vi "SPD.AP Meas Const T.vi"(5 "Continue":refnum<vi>, 6 "Temperature index":i32, 7 "Progress":refnum<vi>, 8 "Error In":errorcluster, 10 "APParams":T1, 11 "SPD.Stand Ctrl in":T2 {"spdDeviceSession"."hidSPD.Sturtup Values"."HV_bias" format="%#_6p, V"; "spdDeviceSession"."hidSPD.Sturtup Values"."TSet" format="%#_6p, DegC"; "spdDeviceSession"."hidSPD.Controller"."HV_bias" format="%#_6p, V"; "spdDeviceSession"."hidSPD.Controller"."TSet" format="%#_6p, DegC"}) -> (0 "Error Out":errorcluster, 1 "pass":bool, 2 "Report":string, 3 "SPD.Stand Ctrl out":T2 {"spdDeviceSession"."hidSPD.Sturtup Values"."HV_bias" format="%#_6p, V"; "spdDeviceSession"."hidSPD.Sturtup Values"."TSet" format="%#_6p, DegC"; "spdDeviceSession"."hidSPD.Controller"."HV_bias" format="%#_6p, V"; "spdDeviceSession"."hidSPD.Controller"."TSet" format="%#_6p, DegC"})   [LabVIEW 2018]
uses:
  typedefs/SPD.Stand Ctrl.ctl
  Instruments/SPD HID Interface/hidSPDLibForLabView/LibVIs/hidSPD Controls/hidSPD Device Session.ctl
  Instruments/SPD HID Interface/hidSPDLibForLabView/LibVIs/hidSPD Controls/hidSPD Controller.ctl
  Instruments/SPD HID Interface/hidSPDLibForLabView/LibVIs/hidSPD Controls/hidSPD SPD Type.ctl
  Instruments/KC705 DevBoard/typedefs/DevB.Session.ctl
  Instruments/KeySight 53230A/typedefs/FreqC.Session.ctl
  Instruments/KeySight 8164B/KeySight 8164B LAN InstrLib/typedefs/KeySight 8164B control.ctl
  Instruments/LeCroy SDA830/typedefs/LeCroy.Session.ctl
  typedefs/SPD.Events.ctl
  ConfigFile/SPD.Config File ctrl.ctl
  <vilib>/Utility/config.llb/Config Data RefNum.ctl
  typedefs/SPD.Meas Result.ctl
  typedefs/SPD.Queues.ctl
  typedefs/SPD.Stand state.ctl
  typedefs/SPD.AP Test Params.ctl
  typedefs/SPD.QE Strobe_Phase Tune Limits.ctl
  Instruments/KeySight 8164B/KeySight 8164B LAN InstrLib.lvlib
  <vilib>/Utility/config.llb/NI_LVConfig.lvlib
  Instruments/SPD HID Interface/hidSPDLibForLabView/hidSPDLibForLabView.lvlib
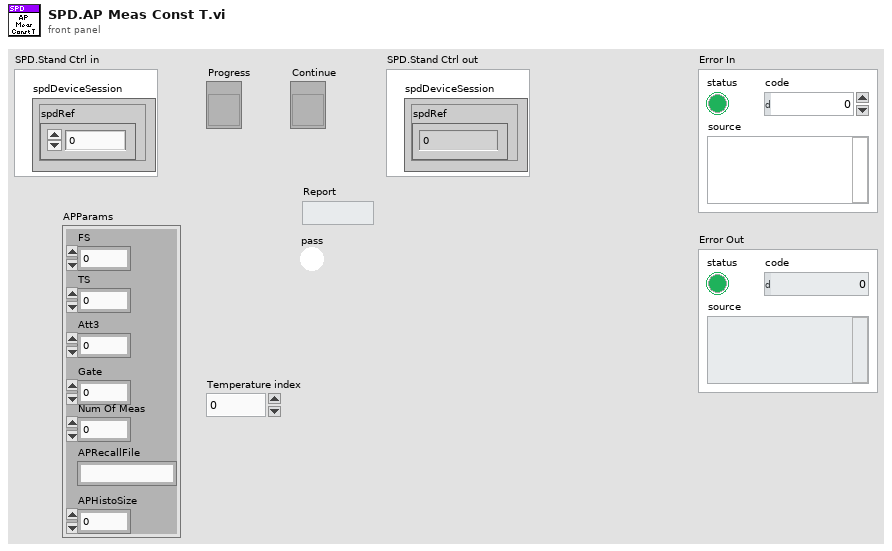
[diagram p1: front panel]
types:
  T1 = typedef "SPD.AP Test Params.ctl" = cluster{"FS":i32, "TS":i32, "Att3":dbl, "Gate":dbl, "Num Of Meas":i32, "APRecallFile":string, "APHistoSize":i32}
  T2 = typedef "SPD.Stand Ctrl.ctl" = cluster{"spdDeviceSession":T3, "DevBSession":T6, "FreqCSession":T7, "8164BSession":T8, "LeCroySession":T9, "Events":T10, "configFile":T11, "SPD.Result":T13, "SPD.Queues":T14, "Console":refnum<vi>}
  T3 = typedef "hidSPDLibForLabView.lvlib/hidSPD Device Session.ctl" = cluster{"spdRef":u64, "connected":bool, "spdName":string, "hidSPD.Controller":T4, "hidSPD.Sturtup Values":T4, "SPD Type":T5}
  T4 = typedef "hidSPDLibForLabView.lvlib/hidSPD Controller.ctl" = cluster{"TSet":sgl, "HV_bias":sgl, "DDS_stb_code":u16}
  T5 = typedef "hidSPDLibForLabView.lvlib/hidSPD SPD Type.ctl" = enum16{"Free Run", "Gate"}
  T6 = typedef "DevB.Session.ctl" = cluster{"DevBRef":refnum<visa-resource-name>, "connected":bool}
  T7 = typedef "FreqC.Session.ctl" = cluster{"FreqCRef":refnum<visa-resource-name>, "timeout":dbl, "Gate":dbl, "connected":bool}
  T8 = typedef "KeySight 8164B LAN InstrLib.lvlib/KeySight 8164B control.ctl" = cluster{"Connection ID":refnum<k5>, "Connected":bool, "Info":string, "Slots Info":string[]}
  T9 = typedef "LeCroy.Session.ctl" = cluster{"LeCroySession":refnum<visa-resource-name>, "connected":bool}
  T10 = typedef "SPD.Events.ctl" = cluster{"DCRTest":refnum<user-event>, "Stop":refnum<user-event>}
  T11 = typedef "SPD.Config File ctrl.ctl" = cluster{"configFile ref":T12, "configFile path":path, "equipmentFile ref":T12}
  T12 = typedef "NI_LVConfig.lvlib/Config Data RefNum.ctl" = refnum<k1>
  T13 = typedef "SPD.Meas Result.ctl" = cluster{"HV_Bias":dbl[][][], "Stb_code":dbl[], "Temprature":dbl[], "Data":dbl[][][][], "DateTime":string}
  T14 = typedef "SPD.Queues.ctl" = cluster{"state queue":refnum<queue>}
  T15 = typedef "SPD.QE Strobe_Phase Tune Limits.ctl" = cluster{"ph_start":i32, "ph_stop":i32, "ph_step":i32}
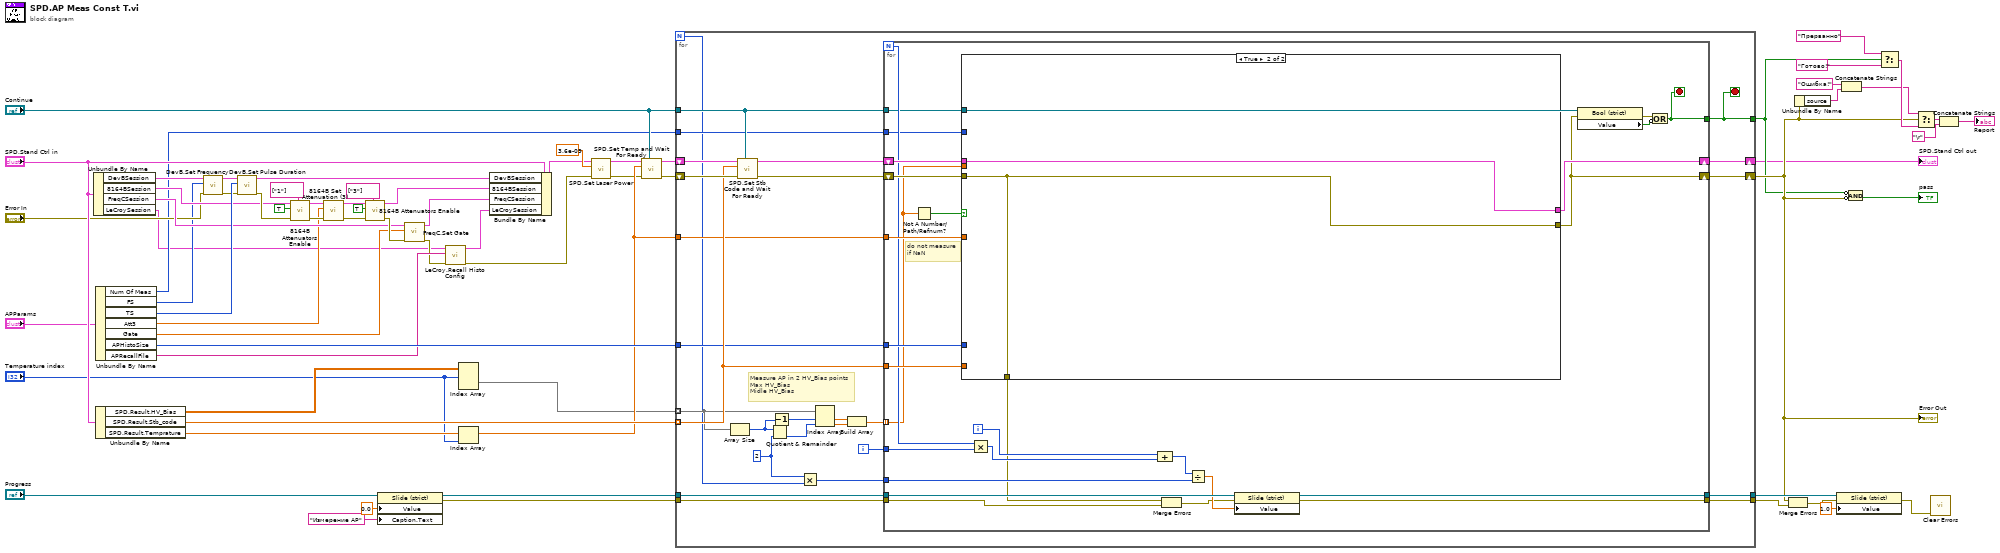
[diagram p0: block diagram]
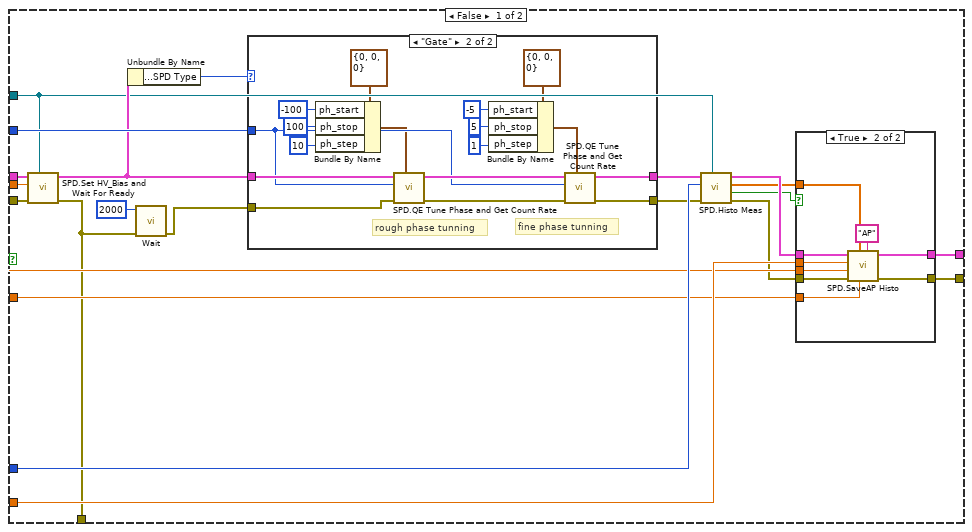
[diagram p2: hidden frame]
diagram:
  n1 = Unbundle By Name("SPD.Stand Ctrl in") -> ("DevBSession"=w61:T6, "8164BSession"=w51:T8, "FreqCSession"=w50:T7, "LeCroySession"=w7:T9)
  n2 = Unbundle By Name("APParams") -> ("Num Of Meas"=w38:i32, "FS"=w36:i32, "TS"=w59:i32, "Att3"=w37:dbl, "Gate"=w39:dbl, "APHistoSize"=w23:i32, "APRecallFile"=w9:string)
  n3 = Unbundle By Name("SPD.Stand Ctrl in") -> ("SPD.Result.HV_Bias"=w62:dbl[][][], "SPD.Result.Stb_code"=w63:dbl[], "SPD.Result.Temprature"=w64:dbl[])
  n4 = call "DevB.Set Frequency.vi"("error in (no error)"="Error In", "Frequency"=w36, "DevB Session in"=w61) -> ("error out"=w58:errorcluster, "DevB Session out"=w60:T6)  [unwired: 7 in]
  n5 = call "DevB.Set Pulse Duration.vi"("error in (no error)"=w58, "Pulse Duration"=w59, "DevB Session in"=w60) -> ("error out"=w53:errorcluster, "DevB Session out"=w49:T6)  [unwired: 7 in]
  n6 = call "8164B Attenuators Enable.vi"("Slots"=string[] ["1"], "error in"=w53, "Enable"=TRUE, "KeySight 8164B control in"=w51) -> ("error out"=w41:errorcluster, "KeySight 8164B control out"=w43:T8)  [unwired: 6 in]
  n7 = call "8164B Set Attenuation (3).vi"("error in"=w41, "Att 3, dB"=w37, "KeySight 8164B control in"=w43) -> ("error out"=w40:errorcluster, "KeySight 8164B control out"=w42:T8)  [unwired: 7 in]
  n8 = call "8164B Attenuators Enable.vi"("Slots"=string[] ["3"], "error in"=w40, "Enable"=TRUE, "KeySight 8164B control in"=w42) -> ("error out"=w52:errorcluster, "KeySight 8164B control out"=w48:T8)  [unwired: 6 in]
  n9 = property class="Slide (strict)"(reference="Progress", "Value"=0.0, "Caption.Text"="Измерение AP") -> (reference out=w15:refnum<vi>, error out=w13:errorcluster)  [unwired: 1 in]
  n10 = call "FreqC.Set Gate.vi"("error In"=w52, "Gate, sec"=w39, "FreqC Session in"=w50) -> ("error out"=w8:errorcluster, "FreqC Session out"=w47:T7)  [unwired: 7 in]
  n11 = call "LeCroy.Recall Histo Config.vi"("Error In"=w8, "Filename (panel.lss)"=w9, "LeCroy.Session in"=w7) -> ("Error Out"=w2:errorcluster, "LeCroy.Session out"=w6:T9)  [unwired: 7 in]
  n12 = Index Array(array=w62, index (dim 0)="Temperature index") -> (element=w18:dbl[][])  [unwired: 2 in]
  n13 = Index Array(array=w64, index="Temperature index") -> (element=w19:dbl)
  n14 = Bundle By Name(cluster="SPD.Stand Ctrl in", "DevBSession"=w49, "8164BSession"=w48, "FreqCSession"=w47, "LeCroySession"=w6) -> (w4:T2)
  n15 = call "SPD.Set Laser Power.vi"("Error In"=w2, "Pset"=3.6e-09, "SPD.Stand Ctrl in"=w4) -> ("Error Out"=w1:errorcluster, "SPD.Stand Ctrl out"=w3:T2)  [unwired: 7 in]
  n16 = call "SPD.Set Temp and Wait For Ready.vi"("Continue"="Continue", "Error In"=w1, "Tset"=w19, "SPD.Stand Ctrl in"=w3) -> ("Error Out"=w21:errorcluster, "SPD.Stand Ctrl out"=w20:T2)  [unwired: 6 in]
  n17 = for {
    N -> [w71]
    tunnel: w18 -> [w84] mode=indexing
    tunnel: w63 -> [w87] mode=indexing
    shift-right: [w95] -> w22
    shift-left: w20 -> [w93]
    shift-right: [w94] -> w26
    shift-left: w21 -> [w92]
    tunnel: "Continue" -> [w77]
    tunnel: [w90] -> w25
    tunnel: w15 -> [w89]
    tunnel: [w88] -> w67
    tunnel: w38 -> [w76]
    tunnel: w23 -> [w86]
    tunnel: w19 -> [w85]
    tunnel: w13 -> [w70]
    tunnel: [w69] -> w11
    i -> [w91]
    stop <- w90 stop-if-true
    w72 = 2 ("y")
    # "Measure AP in 2 HV_Bias points\nMax HV_Bias \nMidle HV_Bias"
    n18 = Array Size(array=w84) -> (size(s)=w82:i32)
    n19 = call "SPD.Set Stb Code and Wait For Ready.vi"("Continue"=w77, "Error In"=w92, "Strobe code"=w87, "SPD.Stand Ctrl in"=w93) -> ("Error Out"=w74:errorcluster, "SPD.Stand Ctrl out"=w75:T2)  [unwired: 6 in]
    n20 = Quotient & Remainder(x=w82, y=w72) -> (floor(x/y)=w83:i32)  [unwired: 1 out]
    n21 = Decrement(x=w82) -> (x-1=w81:i32)
    n22 = Multiply(x=w72, y=w71) -> (x*y=w73:i32)
    n23 = Index Array(array=w84, index #1=w81, index #2=w83) -> (element #1=w80:dbl, element #2=w79:dbl)
    n24 = Build Array(w80, w79) -> (w78:dbl[])
    n25 = for {
      N -> [w105]
      tunnel: w78 -> [w96] mode=indexing
      shift-right: [w108] -> w95
      shift-left: w75 -> [w122]
      shift-right: [w107] -> w94
      shift-left: w74 -> [w121]
      tunnel: w77 -> [w99]
      tunnel: w91 -> [w111]
      tunnel: [w118] -> w90
      tunnel: w89 -> [w117]
      tunnel: w73 -> [w115]
      tunnel: [w113] -> w88
      tunnel: w76 -> [w103]
      tunnel: w87 -> [w109]
      tunnel: w86 -> [w110]
      tunnel: w85 -> [w106]
      tunnel: w70 -> [w101]
      tunnel: [w100] -> w69
      i -> [w104]
      stop <- w118 stop-if-true
      # "do not measure\nif NaN"
      n26 = Not A Number/Path/Refnum?(number/path/refnum=w96) -> (NaN/Path/Refnum?=w97:bool)
      n27 = case shown="True" w97 {
        tunnel: w122 -> [w143 w175]
        tunnel: w121 -> [w142 w174]
        tunnel: w110 -> [w141 _]
        tunnel: w109 -> [w140 _]
        tunnel: w96 -> [w139 _]
        tunnel: [w138 w175] -> w108
        tunnel: [w137 w174] -> w107
        tunnel: w106 -> [w136 _]
        tunnel: w103 -> [w130 _]
        tunnel: w99 -> [w127 _]
        tunnel: [w125 w174] -> w98
        frame False {
          n28 = call "SPD.Set HV_Bias and Wait For Ready.vi"("Continue"=w127, "Error In"=w142, "HV_Bias"=w139, "SPD.Stand Ctrl in"=w143) -> ("Error Out"=w125:errorcluster, "SPD.Stand Ctrl out"=w129:T2)  [unwired: 6 in]
          n29 = Unbundle By Name(w129) -> ("spdDeviceSession.SPD Type"=w128:T5)
          n30 = call "Wait.vi"("error in (no error)"=w125, "milliseconds to wait"=u32 2000) -> ("error out"=w124:errorcluster)  [unwired: 9 in]
          n31 = case shown="\"Gate\"" w128 {
            tunnel: [w156 w168] -> w135
            tunnel: [w155 w167] -> w134
            tunnel: w129 -> [w156 w166]
            tunnel: w130 -> [_ w159]
            tunnel: w124 -> [w155 w157]
            frame "Free Run", Default {
            }
            frame "Gate" {
              # "fine phase tunning"
              # "rough phase tunning"
              n32 = Bundle By Name(cluster=T15 {"ph_start"=0, "ph_stop"=0, "ph_step"=0} ("SPD.QE Strobe_Phase Tune Limits"), "ph_start"=-100, "ph_stop"=100, "ph_step"=10) -> (w158:T15)
              n33 = call "SPD.QE Tune Phase and Get Count Rate.vi"("SPD.QE Strobe_Phase Tune Limits"=w158, "Error In"=w157, "Num of FreqC Meas"=w159, "SPD.Stand Ctrl in"=w166) -> ("Error Out"=w164:errorcluster, "SPD.Stand Ctrl out"=w165:T2)  [unwired: 4 in, 2 out]
              n34 = Bundle By Name(cluster=T15 {"ph_start"=0, "ph_stop"=0, "ph_step"=0} ("SPD.QE Strobe_Phase Tune Limits"), "ph_start"=-5, "ph_stop"=5, "ph_step"=1) -> (w172:T15)
              n35 = call "SPD.QE Tune Phase and Get Count Rate.vi"("SPD.QE Strobe_Phase Tune Limits"=w172, "Error In"=w164, "Num of FreqC Meas"=w159, "SPD.Stand Ctrl in"=w165) -> ("Error Out"=w167:errorcluster, "SPD.Stand Ctrl out"=w168:T2)  [unwired: 4 in, 2 out]
            }
          }
          n36 = call "SPD.Histo Meas.vi"("Continue"=w127, "Error In"=w134, "Histo length"=w141, "SPD.Stand Ctrl in"=w135) -> ("Error Out"=w131:errorcluster, "pass"=w126:bool, "Histo"=w132:dbl[], "SPD.Stand Ctrl out"=w133:T2)  [unwired: 4 in]
          n37 = case shown="True" w126 {
            tunnel: w140 -> [_ w154]
            tunnel: w139 -> [_ w153]
            tunnel: [w145 w152] -> w138
            tunnel: [w144 w151] -> w137
            tunnel: w136 -> [_ w150]
            tunnel: w133 -> [w145 w149]
            tunnel: w132 -> [_ w148]
            tunnel: w131 -> [w144 w147]
            frame False {
            }
            frame True {
              n38 = call "SPD.SaveAP Histo.vi"("Name"="AP", "Temperature"=w150, "AP Histo"=w148, "Error In"=w147, "HV_bias"=w153, "Stb_Code"=w154, "SPD.Stand Ctrl in"=w149) -> ("Error Out"=w151:errorcluster, "SPD.Stand Ctrl out"=w152:T2)  [unwired: 3 in]
            }
          }
        }
        frame True {
        }
      }
      n39 = Multiply(x=w105, y=w111) -> (x*y=w112:i32)
      n40 = Compound Arithmetic op=ADD(w104, w112) -> (w116:i32)
      n41 = Merge Errors(w98, w101) -> (w102:errorcluster)
      n42 = Divide(x=w116, y=w115) -> (x/y=w114:dbl)
      n43 = property class="Slide (strict)"(reference=w117, error in=w102, "Value"=w114) -> (reference out=w113:refnum<vi>, error out=w100:errorcluster)
      n44 = property class="Bool (strict)"(reference=w99, error in=w107) -> (error out=w119:errorcluster, "Value"=w120:bool)  [unwired: 1 out]
      n45 = Compound Arithmetic op=OR(w119, invert w120) -> (w118:bool)
    }
  }
  "SPD.Stand Ctrl out" <- w22
  "Error Out" <- w26
  n46 = Merge Errors(w26, w11) -> (w12:errorcluster)
  n47 = Unbundle By Name(w26) -> ("source"=w31:string)
  n48 = property class="Slide (strict)"(reference=w67, error in=w12, "Value"=1.0) -> (error out=w65:errorcluster)  [unwired: 1 out]
  n49 = Concatenate Strings("Ошибка!" ("t"), w31) -> (w32:string)
  n50 = Compound Arithmetic op=AND(invert w25, invert w26) -> (→"pass":bool)
  n51 = Select(t="Прерванно" ("Report"), s=w25, f="Готово!") -> (s? t:f=w34:string)
  n52 = Select(t=w32, s=w26, f=w34) -> (s? t:f=w29:string)
  n53 = call <vilib>:"Clear Errors.vi"("error in (no error)"=w65) -> ()  [unwired: 5 in, 2 out]
  n54 = Concatenate Strings(w29, "\r") -> (→"Report":string)
